vi "Get Rx Error Channel References.vi"(8 "error in":errorcluster, 11 "status reference in":T1=18446744073709551615 format="%.0x") -> (0 "error out":errorcluster, 1 "Rx specific error count references":T2 {"timeout" format="%.0x"; "bit timing" format="%.0x"; "long word" format="%.0x"; "parity" format="%.0x"; "gap" format="%.0x"}, 2 "Rx error count reference":T1 format="%.0x", 3 "status reference out":T1 format="%.0x")   [LabVIEW 2020, in "Ballard ARINC 429 Scripting.lvlib"]
uses:
  <vilib>/NI VeriStand/Custom Device API/Custom Device Item Ref.ctl
  Ballard ARINC 429 Scripting.lvlib
  <vilib>/NI VeriStand/Custom Device Tools/Custom Device Utility Library/Custom Device Utility Library.lvlib
  <vilib>/NI VeriStand/Custom Device Tools/Custom Device Utility Library/NI VeriStand - Search for Item by Name.vi
  Constants.vi
  <vilib>/NI VeriStand/Custom Device API/Custom Device API.lvlib
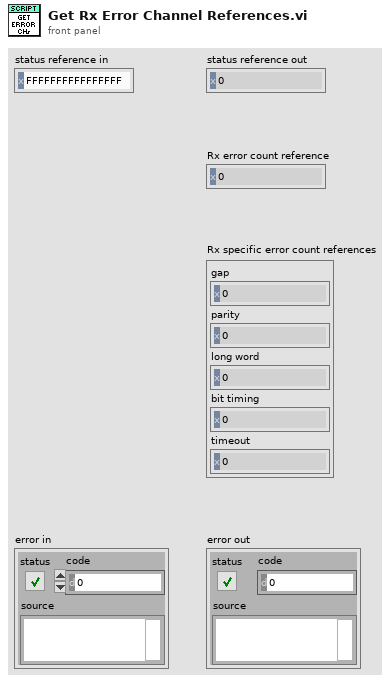
[diagram p1: front panel]
types:
  T1 = typedef "Custom Device API.lvlib/Custom Device Item Ref.ctl" = u64
  T2 = cluster{"gap":T1, "parity":T1, "long word":T1, "bit timing":T1, "timeout":T1}
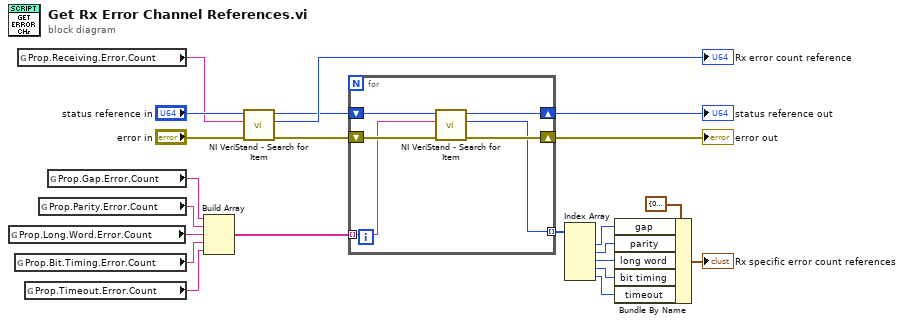
[diagram p0: block diagram]
diagram:
  n1 = global read "Constants.vi" "Prop.Long.Word.Error.Count"() -> (w12:string)
  n2 = global read "Constants.vi" "Prop.Bit.Timing.Error.Count"() -> (w11:string)
  n3 = global read "Constants.vi" "Prop.Receiving.Error.Count"() -> (w19:string)
  n4 = global read "Constants.vi" "Prop.Timeout.Error.Count"() -> (w10:string)
  n5 = global read "Constants.vi" "Prop.Parity.Error.Count"() -> (w13:string)
  n6 = global read "Constants.vi" "Prop.Gap.Error.Count"() -> (w14:string)
  n7 = Build Array(w14, w13, w12, w11, w10) -> (w9:string[])
  n8 = call-poly <vilib>:"NI VeriStand - Search for Item.vi"("error in"="error in", "Item Name"=w19, "Section Ref in"="status reference in") -> ("error out"=w17:errorcluster, "Item Ref"=→"Rx error count reference":T1, "Section Ref out"=w18:T1)  [unwired: 5 in, 1 out]
  n9 = for {
    shift-right: [w25] -> w15
    shift-left: w18 -> [w28]
    shift-right: [w26] -> w16
    shift-left: w17 -> [w27]
    tunnel: w9 -> [w24] mode=indexing
    tunnel: [w23] -> w8 mode=indexing
    n10 = call-poly <vilib>:"NI VeriStand - Search for Item.vi"("error in"=w27, "Item Name"=w24, "Section Ref in"=w28) -> ("error out"=w26:errorcluster, "Item Ref"=w23:T1, "Section Ref out"=w25:T1)  [unwired: 5 in, 1 out]
  }
  "error out" <- w16
  "status reference out" <- w15
  n11 = Index Array(array=w8) -> (element #1=w5:T1, element #2=w4:T1, element #3=w6:T1, element #4=w3:T1, element #5=w2:T1)  [unwired: 5 in]
  n12 = Bundle By Name(cluster=T2 {"gap"=0, "parity"=0, "long word"=0, "bit timing"=0, "timeout"=0} ("Rx specific error count references"), "gap"=w5, "parity"=w4, "long word"=w6, "bit timing"=w3, "timeout"=w2) -> (→"Rx specific error count references":T2)
